vi "SQL_CreateTable.vi"(8 "error in (no error)":errorcluster, 9 "column info":T1[](array[typedef]), 10 "Table Name":string, 11 "SQL in":refnum<class "SQL.lvclass">) -> (0 "error out":errorcluster, 3 "SQL out":refnum<class "SQL.lvclass">)   [LabVIEW 2012, in "SQL.lvclass"]
uses:
  SQL.lvclass
  <vilib>/addons/database/Auxilliary.llb/DB Tools Column Info.ctl
  <vilib>/addons/database/Auxilliary.llb/DB Tools DataTypes.ctl
  <vilib>/addons/database/NI_Database_API.lvlib
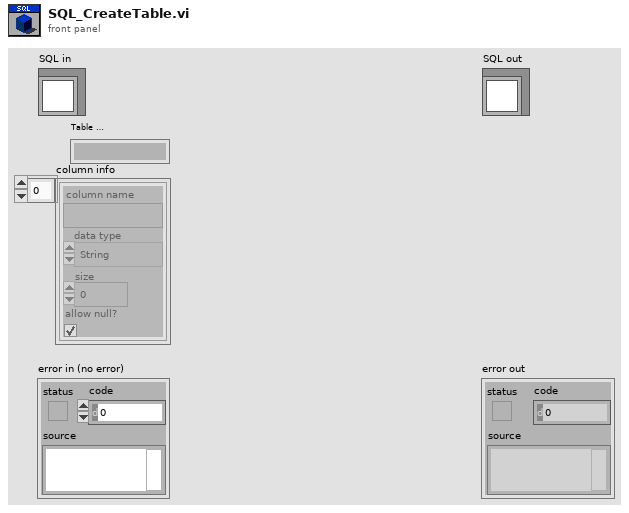
[diagram p1: front panel]
types:
  T1 = typedef "NI_Database_API.lvlib/DB Tools Column Info.ctl" = cluster{"column name":string, "data type":T2, "size":i32, "allow null?":bool}
  T2 = typedef "NI_Database_API.lvlib/DB Tools DataTypes.ctl" = enum16{"String", "Long (I32)", "Single (SGL)", "Double (DBL)", "Date/Time", "Binary"}
  T3 = typedef "SQL.lvclass/ObjectAttributes.ctl" = cluster{"DB Connection Reference":T4}
  T4 = typedef "NI_Database_API.lvlib/Conn ObjectReference.ctl" = refnum<k1>
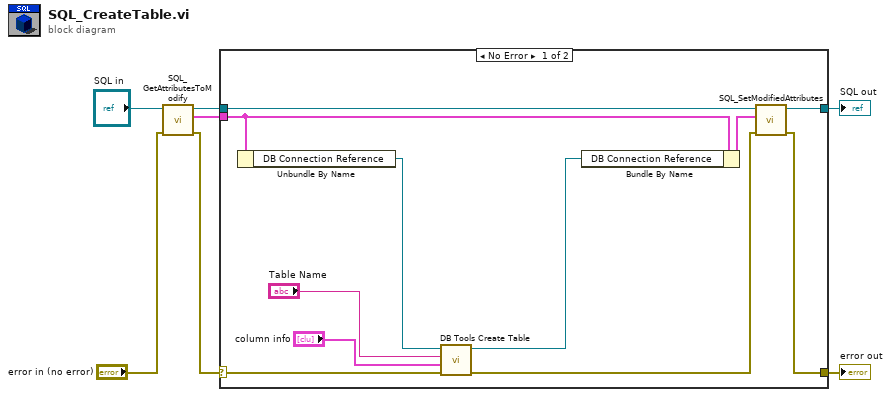
[diagram p0: block diagram]
diagram:
  n1 = call "SQL_GetAttributesToModify.vi"("error in (no error)"="error in (no error)", "reference in"="SQL in") -> ("error out"=w2:errorcluster, "Attributes"=w1:T3, "reference out"=w4:refnum<class "SQL.lvclass">)  [unwired: 6 in, 1 out]
  n2 = case shown="No Error" w2 {
    selector: w2 -> [w18 w20]
    tunnel: [w14 w20] -> w7
    tunnel: [w16 w19] -> w6
    tunnel: w4 -> [w17 w19]
    tunnel: w1 -> [w12 _]
    frame No Error {
      n3 = Unbundle By Name(w12) -> ("DB Connection Reference"=w13:T4)
      n4 = call <vilib>:"DB Tools Create Table.vi"("error in (no error)"=w18, "column information"="column info", "table"="Table Name", "connection reference"=w13) -> ("error out"=w15:errorcluster, "connection reference out"=w10:T4)  [unwired: 4 in]
      n5 = Bundle By Name(cluster=w12, "DB Connection Reference"=w10) -> (w11:T3)
      n6 = call "SQL_SetModifiedAttributes.vi"("error in (no error)"=w15, "Attributes"=w11, "reference in"=w17) -> ("error out"=w14:errorcluster, "reference out"=w16:refnum<class "SQL.lvclass">)  [unwired: 7 in]
    }
    frame Error {
    }
  }
  "error out" <- w7
  "SQL out" <- w6
